vi "Make Node.vi"(8 "error in (no error)":errorcluster, 10 "Node Name":string, 11 "CI Deserializer in":refnum<class "CI Deserializer.lvclass">) -> (0 "error out":errorcluster, 2 "Node Reference":refnum<data-value>, 3 "CI Deserializer out":refnum<class "CI Deserializer.lvclass">)   [LabVIEW 2014, in "CI Deserializer.lvclass"]
uses:
  CI Deserializer.lvclass
  <vilib>/ni/Configuration Framework/Node/NISE_CEF_Node.lvclass
  <vilib>/ni/Configuration Framework/class discovery singleton/class discovery singleton methods.ctl
  Serializable Node/Serializable Node.lvclass
  <vilib>/ni/Configuration Framework/class discovery singleton/class discovery singleton.lvlib
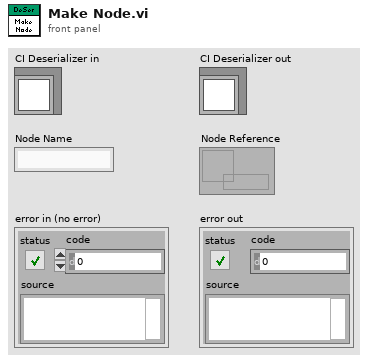
[diagram p1: front panel]
types:
  T1 = typedef "class discovery singleton.lvlib/class discovery singleton methods.ctl" = enum16{"add search paths", "load class by name", "list available classes", "get class path", "delete cache"}
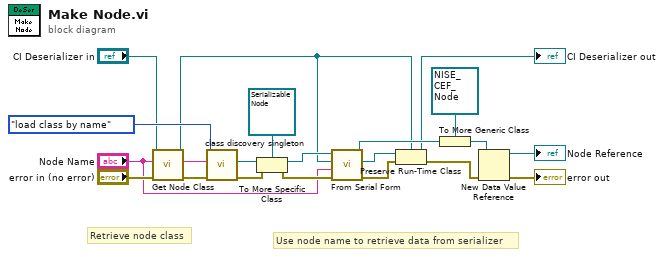
[diagram p0: block diagram]
diagram:
  # "Retrieve node class"
  # "Use node name to retrieve data from serializer"
  n1 = call-dynamic "Get Node Class.vi"("error in (no error)"="error in (no error)", "Node Name"="Node Name", "CI Deserializer in"="CI Deserializer in") -> ("error out"=w3:errorcluster, "Node Class"=w2:string, "CI Deserializer out"=w5:refnum<class "CI Deserializer.lvclass">)  [unwired: 6 in]
  n2 = call <vilib>:"class discovery singleton.vi"("error in"=w3, "Class Name"=w2, "method"=class_discovery_singleton_methods."load class by name") -> ("error out"=w12:errorcluster, "LabVIEW Object"=w10:refnum<class>)  [unwired: 5 in, 2 out]
  n3 = To More Specific Class(target class=refnum<class "Serializable Node.lvclass"> refnum ("Serializable Node.lvclass"), reference=w10, error in=w12) -> (specific class reference=w14:refnum<class "Serializable Node.lvclass">, error out=w13:errorcluster)
  n4 = call-dynamic "From Serial Form.vi"("error in (no error)"=w13, "Node"="Node Name", "CI Deserializer in"=w5, "Serializable Node in"=w14) -> ("error out"=w16:errorcluster, "CI Deserializer out"=w15:refnum<class "CI Deserializer.lvclass">, "Serializable Node out"=w18:refnum<class "Serializable Node.lvclass">)  [unwired: 5 in]
  n5 = Preserve Run-Time Class(object in=w15, error in=w16, 2:w5) -> (object out=→"CI Deserializer out":refnum<class "CI Deserializer.lvclass">, error out=w17:errorcluster)
  n6 = To More Generic Class(target class=refnum<class "NISE_CEF_Node.lvclass"> refnum ("NISE_CEF_Node"), reference=w18) -> (generic class reference=w20:refnum<class "NISE_CEF_Node.lvclass">)
  n7 = New Data Value Reference(data value=w20, error in=w17) -> (data value reference=→"Node Reference":refnum<data-value>, error out=→"error out":errorcluster)
